vi "Run Test.vi"(8 "error in (no error)":errorcluster, 11 "Test Template in":refnum<class "Power On Driver.lvclass">) -> (0 "error out":errorcluster, 1 "Positions":i32[](array[numeric]), 2 "Tests Passed":bool[](array[boolean]), 3 "Test Template out":refnum<class "Power On Driver.lvclass">, 5 "Fail Codes":string[](array[string]))   [LabVIEW 2015, in "Power On Driver.lvclass"]
uses:
  Power On Driver.lvclass
  Test Class/Test Class.lvclass
  Classes/Application/Class/Application.lvclass
  Driver Test/Driver Test.lvclass
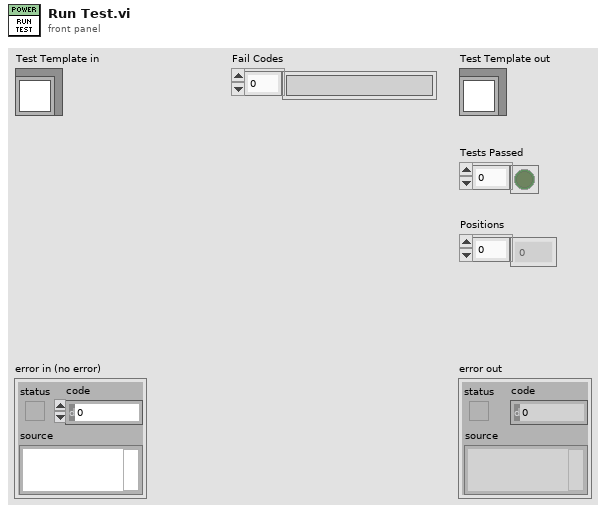
[diagram p1: front panel]
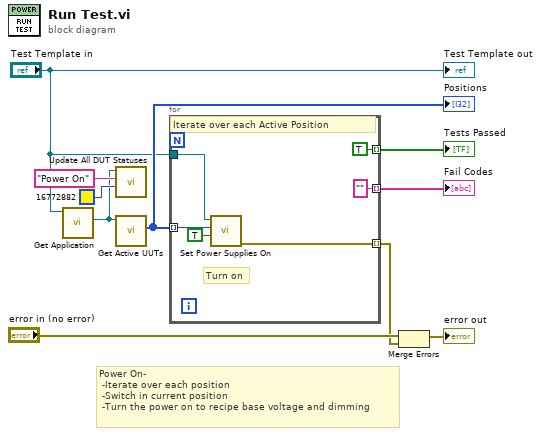
[diagram p0: block diagram]
diagram:
  # "Power On-\n\t-Iterate over each position\n\t-Switch in current position\n\t-Turn the power on to recipe base voltage and dimming"
  n1 = call "Get Application.vi"("Test Class in"="Test Template in") -> ("Application.lvlib:Application.lvclass"=w4:refnum<class "Application.lvclass">)  [unwired: 9 in, 1 out]
  n2 = call "Update All DUT Statuses.vi"("BG Color"=u32 16772882, "Message ('')"="Power On", "Application in"=w4) -> ()  [unwired: 7 in, 2 out]
  n3 = call "Get Active UUTs.vi"("Application in"=w4) -> ("Active Positions"=w6:u32[])  [unwired: 8 in, 2 out]
  "Positions" <- w6
  n4 = for {
    tunnel: w6 -> [w16] mode=indexing
    tunnel: [w14] -> w7 mode=indexing
    tunnel: "Test Template in" -> [w13]
    tunnel: [TRUE] -> w2 mode=indexing
    tunnel: [""] -> w1 mode=indexing
    # "Turn on"
    # "Iterate over each Active Position"
    n5 = call "Set Power Supplies On.vi"("Power On"=TRUE, "Active Positions"=w16, "Driver Test"=w13) -> ("error out"=w14:errorcluster)  [unwired: 8 in]
  }
  "Tests Passed" <- w2
  "Fail Codes" <- w1
  n6 = Merge Errors("error in (no error)", w7) -> (→"error out":errorcluster)
  "Test Template out" <- "Test Template in"
